vi "Append Report Text (str).vi"(0 "report in":refnum<class "NI_Excel.lvclass">, 1 "MS Office parameters":T1, 2 "format string (%.3f)":string="%.3f", 7 "text":string, 9 "append on new line? (F)":bool, 11 "error in (no error)":errorcluster) -> (4 "report out":refnum<class "NI_Excel.lvclass">, 8 "start out (Word)":i32, 10 "end out (Word)":i32, 15 "error out":errorcluster)   [LabVIEW 2020, in "NI_Excel.lvclass"]
doc: "Appends text to the selected report."
uses:
  <vilib>/Utility/NIReport.llb/Excel/NI_Excel.lvclass
  <vilib>/Utility/NIReport.llb/Excel/NI_Excel.lvclass/NI_Excel.ctl
  <vilib>/addons/_office/NI_ReportGenerationToolkit.lvlib
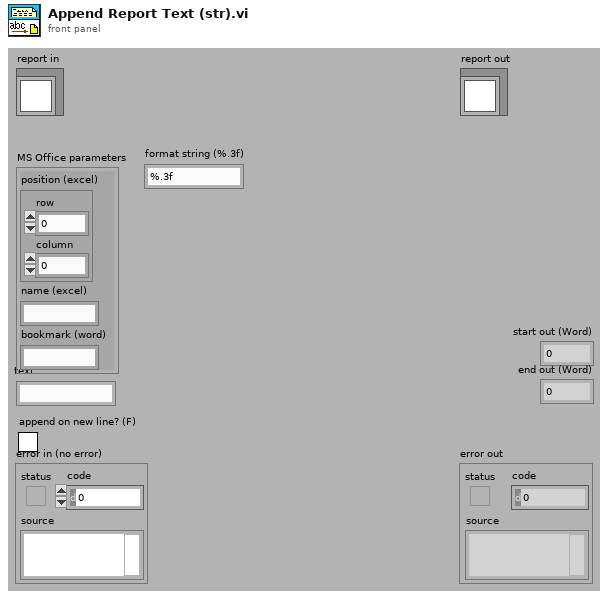
[diagram p1: front panel]
types:
  T1 = cluster{"position (excel)":cluster{"row":i32, "column":i32}, "name (excel)":string, "bookmark (word)":string}
  T2 = typedef "NI_ReportGenerationCore.lvlib/Report Data Members.ctl" = cluster{"font":T3, "from template?":bool}
  T3 = typedef "NI_ReportGenerationCore.lvlib/font.ctl" = cluster{"font name":string, "font size":dbl, "bold":u16, "italic":u16, "underline":u16, "strike through":u16, "font color":u32}
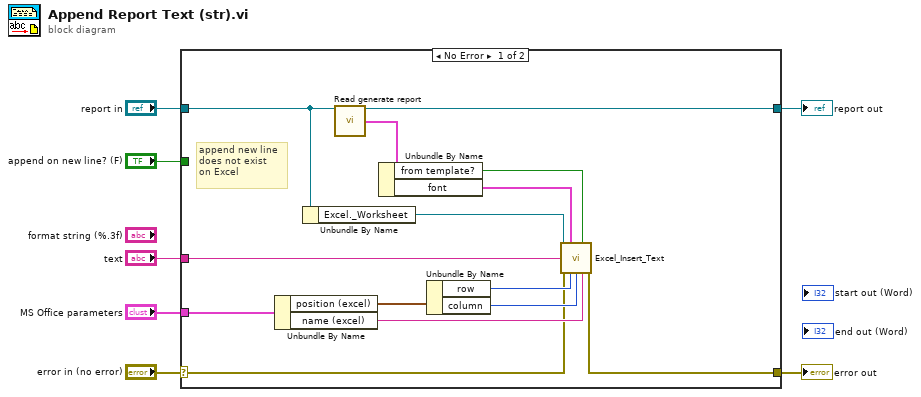
[diagram p0: block diagram]
diagram:
  n1 = case shown="No Error" "error in (no error)" {
    selector: "error in (no error)" -> [w14 w23]
    tunnel: [w13 w23] -> w6
    tunnel: [w11 w22] -> w4
    tunnel: "report in" -> [w12 w22]
    tunnel: "append on new line? (F)" -> [_ _]
    tunnel: "MS Office parameters" -> [w16 _]
    tunnel: "text" -> [w15 _]
    frame No Error {
      # "append new line\ndoes not exist\non Excel"
      n2 = Unbundle By Name(w16) -> ("position (excel)"=w17:cluster{"row":i32, "column":i32}, "name (excel)"=w18:string)
      n3 = Unbundle By Name(w12) -> ("Excel._Worksheet"=w21:refnum<k7>)
      n4 = call-dynamic "Read generate report.vi"("report in"=w12) -> ("report out"=w11:refnum<class "NI_Excel.lvclass">, "generate report"=w10:T2)  [unwired: 12 in, 1 out]
      n5 = Unbundle By Name(w10) -> ("from template?"=w9:bool, "font"=w8:T3)
      n6 = Unbundle By Name(w17) -> ("row"=w20:i32, "column"=w19:i32)
      n7 = call <vilib>:"Excel_Insert_Text.vi"("worksheet"=w21, "font"=w8, "from template?"=w9, "value"=w15, "error in (no error)"=w14, "row"=w20, "column"=w19, "name"=w18) -> ("error out"=w13:errorcluster)  [unwired: 7 out]
    }
    frame Error {
    }
  }
  "error out" <- w6
  "report out" <- w4
